vi "Halt BatchD.vi"() -> ()   [LabVIEW 2017]
panel:
  in  "Halt":bool
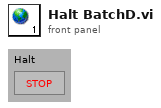
[diagram p1: front panel]
diagram:
